vi "Get Database.vi"(8 "error in (no error)":errorcluster, 11 "Login in":refnum<class "Login.lvclass">) -> (0 "error out":errorcluster, 2 "Database":refnum<class "Database.lvclass">, 3 "Login out":refnum<class "Login.lvclass">)   [LabVIEW 2015, in "Login.lvclass"]
uses:
  Login.lvclass
  API/_Database/Database.lvclass
  Login.lvclass/Login.ctl
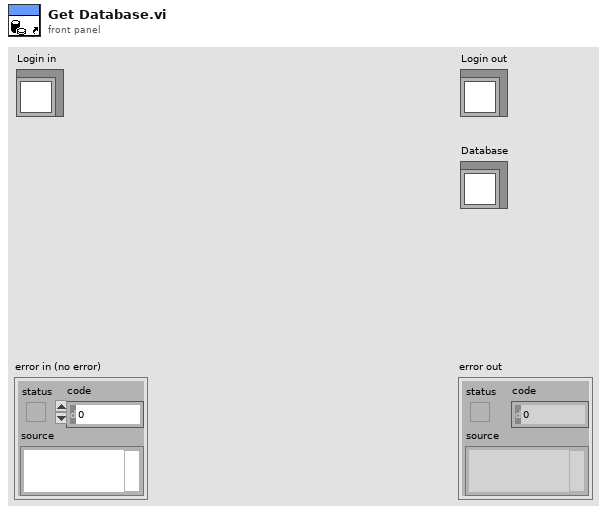
[diagram p1: front panel]
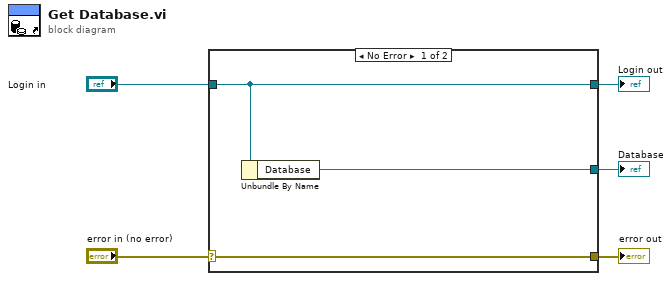
[diagram p0: block diagram]
diagram:
  n1 = case shown="No Error" "error in (no error)" {
    selector: "error in (no error)" -> [w8 w9]
    tunnel: [w8 w9] -> w4
    tunnel: [w7 w10] -> w2
    tunnel: "Login in" -> [w7 w10]
    tunnel: [w6 _] -> w1
    frame No Error {
      n2 = Unbundle By Name(w7) -> ("Database"=w6:refnum<class "Database.lvclass">)
    }
    frame Error {
    }
  }
  "error out" <- w4
  "Login out" <- w2
  "Database" <- w1
